vi "SGUI Set Multiple Reals By Label.vi"(6 "error in":errorcluster, 8 "labels (empty)":string, 9 "format (empty)":string, 10 "numbers (empty)":dbl[](array[numeric])) -> (7 "error out":errorcluster, 11 "control references out":refnum<vi>[](array[refnum]))   [LabVIEW 2020, in "varilib.lvlib"]
doc: "This VI sets value(s) and format(s) of numeric controls designated by label(s) name string. Multiple can be assigned at once by using multiline string 'labels'. One line per control. If empty format string is entered, format stays unchanged. If empty values array is entered, no value is modified. If multiple controls are assigned but just one number or format string is assigned, the same format or/and value is written to all controls.\nNote: NaN numeric value is ignored - it is used as no modify value!\n\nThi VI ignores input errors (will execute anyway) however will generate error if any of the named controls is not found or writting to it fails (invalid type of control)."
uses:
  varilib.lvlib
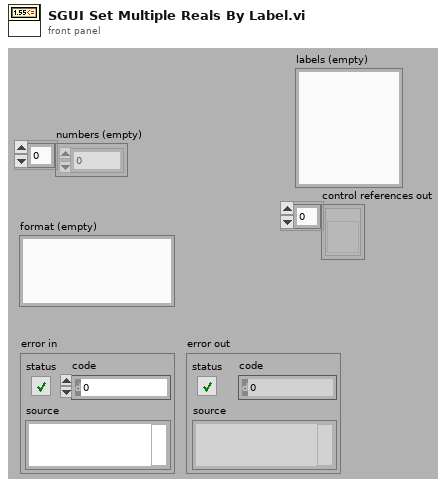
[diagram p1: front panel]
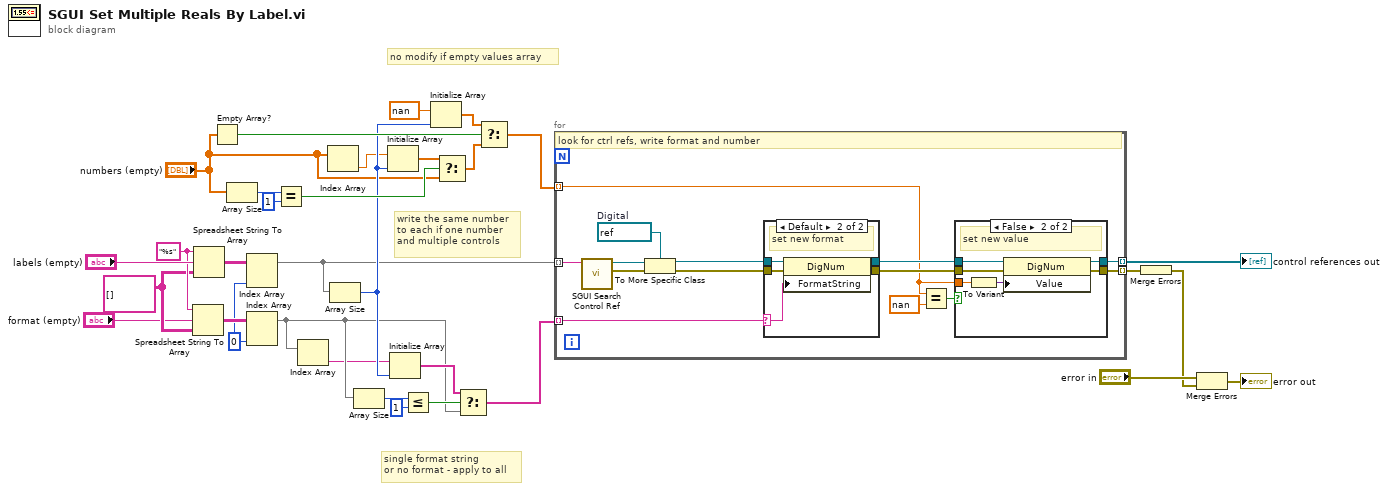
[diagram p0: block diagram]
diagram:
  w3 = 0 ("disabled index (col)")
  w25 = string[][] []
  w26 = "%s"
  # "write the same number\nto each if one number\nand multiple controls"
  # "no modify if empty values array"
  # "single format string\nor no format - apply to all"
  n1 = Spreadsheet String To Array(format string=w26, spreadsheet string="format (empty)", array type (2D Dbl)=w25) -> (array=w22:string[][])  [unwired: 1 in]
  n2 = Spreadsheet String To Array(format string=w26, spreadsheet string="labels (empty)", array type (2D Dbl)=w25) -> (array=w20:string[][])  [unwired: 1 in]
  n3 = Empty Array?(array="numbers (empty)") -> (empty?=w16:bool)
  n4 = Array Size(array="numbers (empty)") -> (size(s)=w13:i32)
  n5 = Index Array(array=w20, index (col)=w3) -> (element=w4:string[])  [unwired: 1 in]
  n6 = Index Array(array=w22, index (col)=w3) -> (element=w2:string[])  [unwired: 1 in]
  n7 = Equal?(x=w13, y=1) -> (x = y?=w10:bool)
  n8 = Index Array(array=w2) -> (element=w1:string)  [unwired: 1 in]
  n9 = Index Array(array="numbers (empty)") -> (element=w7:dbl)  [unwired: 1 in]
  n10 = Array Size(array=w4) -> (size(s)=w8:i32)
  n11 = Array Size(array=w2) -> (size(s)=w24:i32)
  n12 = Initialize Array(w7, w8) -> (w9:dbl[])
  n13 = Initialize Array(w1, w8) -> (w19:string[])
  n14 = Less Or Equal?(x=w24, y=1) -> (x <= y?=w17:bool)
  n15 = Initialize Array(nan, w8) -> (w15:dbl[])
  n16 = Select(t=w9, s=w10, f="numbers (empty)") -> (s? t:f=w11:dbl[])
  n17 = Select(t=w19, s=w17, f=w2) -> (s? t:f=w18:string[])
  n18 = Select(t=w15, s=w16, f=w11) -> (s? t:f=w5:dbl[])
  n19 = for {
    tunnel: w4 -> [w46] mode=indexing
    tunnel: [w41] -> w31 mode=indexing
    tunnel: [w42] -> w32 mode=indexing
    tunnel: w18 -> [w45] mode=indexing
    tunnel: w5 -> [w39] mode=indexing
    w33 = refnum<vi> refnum  # Digital
    # "look for ctrl refs, write format and number"
    n20 = call "SGUI Search Control Ref.vi"("control label (empty)"=w46) -> ("error out"=w37:errorcluster, "control ref out"=w34:refnum<vi>)  [unwired: 8 in, 1 out]
    n21 = To More Specific Class(target class=w33, reference=w34, error in=w37) -> (specific class reference=w35:refnum<vi>, error out=w36:errorcluster)
    n22 = case shown="Default" w45 {
      selector: w45 -> [_ w57]
      tunnel: w36 -> [w56 w61]
      tunnel: [w56 w60] -> w44
      tunnel: [w55 w59] -> w43
      tunnel: w35 -> [w55 w58]
      frame "" {
      }
      frame Default {
        # "set new format"
        n23 = property class="DigNum"(reference=w58, error in=w61, "FormatString"=w57) -> (reference out=w59:refnum<vi>, error out=w60:errorcluster)
      }
    }
    n24 = Equal?(x=w39, y=nan) -> (x = y?=w40:bool)
    n25 = case shown="False" w40 {
      tunnel: w44 -> [w48 w54]
      tunnel: [w48 w53] -> w42
      tunnel: [w47 w52] -> w41
      tunnel: w43 -> [w47 w51]
      tunnel: w39 -> [_ w49]
      frame True {
      }
      frame False {
        # "set new value"
        n26 = To Variant(anything=w49) -> (Variant=w50:variant)
        n27 = property class="DigNum"(reference=w51, error in=w54, "Value"=w50) -> (reference out=w52:refnum<vi>, error out=w53:errorcluster)
      }
    }
  }
  "control references out" <- w31
  n28 = Merge Errors(w32) -> (w27:errorcluster)
  n29 = Merge Errors("error in", w27) -> (→"error out":errorcluster)
